vi "Side.vi"(1 "PicAjust":T1={"TranslationVector"=[], "scale"=2.0, "Pitch（x) "=0.0, "Yaw（y)"=0.0, "Roll（z) "=0.0} {"Roll（z)" scale=-90.0..90.0; "Yaw（y)" scale=-90.0..90.0; "Pitch（x)" scale=-90.0..90.0}, 2 "Input":dbl[](array[numeric])) -> (0 "输出簇":cluster{"x":dbl, "y":dbl})   [LabVIEW 2014]
doc: "轴测图"
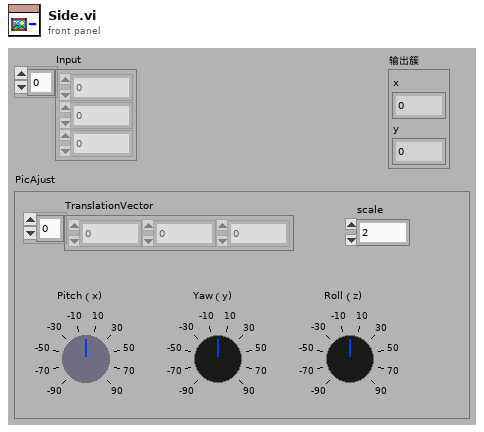
[diagram p1: front panel]
types:
  T1 = cluster{"TranslationVector":dbl[], "scale":dbl, "Pitch（x) ":dbl, "Yaw（y)":dbl, "Roll（z) ":dbl}
  T2 = typedef "NI_Kinematics.lvlib/Quaternion.ctl" = dbl[]
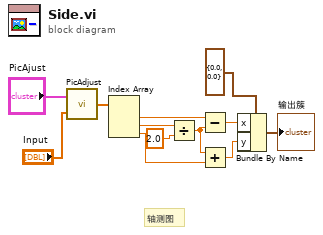
[diagram p0: block diagram]
diagram:
  # "轴测图"
  n1 = call "PicAdjust.vi"("Input"="Input", "PicAjust"="PicAjust") -> ("子数组"=w1:T2)
  n2 = Index Array(array=w1) -> (element #1=w10:dbl, element #2=w12:dbl, element #3=w8:dbl)  [unwired: 3 in]
  n3 = Divide(x=w12, y=2.0) -> (x/y=w9:dbl)
  n4 = Subtract(x=w10, y=w9) -> (x-y=w7:dbl)
  n5 = Add(x=w9, y=w8) -> (x+y=w6:dbl)
  n6 = Bundle By Name(cluster=cluster{"x":dbl, "y":dbl} {"x"=0.0, "y"=0.0} ("Point"), "x"=w7, "y"=w6) -> (→"输出簇":cluster{"x":dbl, "y":dbl})
